vi "Execute Statement.vi"(6 "Values in":string[](array[string]), 8 "error in (no error)":errorcluster, 9 "Parameters in":string[](array[string]), 10 "Statement index in":u64, 11 "IDatabase in":refnum<class "IDatabase.lvclass">) -> (0 "error out":errorcluster, 2 "Result":string[][](array[string]), 3 "IDatabase out":refnum<class "IDatabase.lvclass">)   [LabVIEW 2020, in "IDatabase.lvlib" / "IDatabase.lvclass"]
uses:
  IDatabase.lvclass
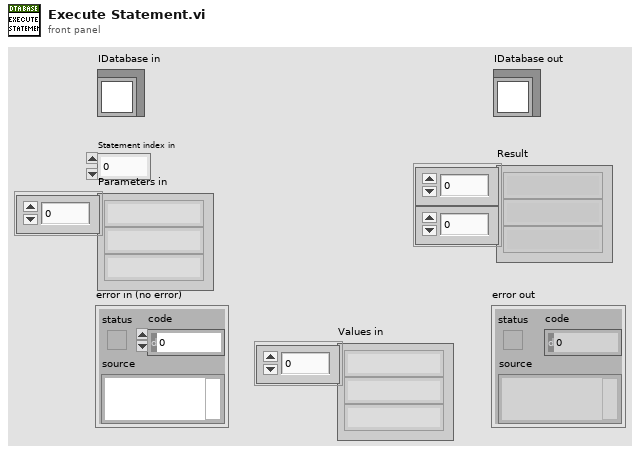
[diagram p1: front panel]
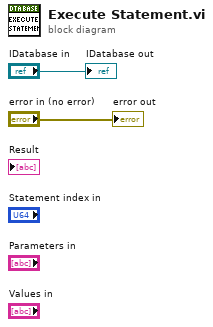
[diagram p0: block diagram]
diagram:
  "error out" <- "error in (no error)"
  "IDatabase out" <- "IDatabase in"
